vi "Graph_manipulations.vi"(0 "RF Slider in":cluster{i32, i32}, 1 "RF Slider 1":cluster{i32, i32}, 2 "Gaussian Noise SD":dbl, 5 "Array in":dbl[](array[numeric]), 7 "AFP Slider":cluster{i32, i32}, 9 "Zero ensemble in":dbl[](array[numeric]), 12 "rho+ in":dbl[](array[numeric]), 13 "rho0 in":dbl[](array[numeric]), 14 "rho- in":dbl[](array[numeric])) -> (4 "Q Graph":cluster{"Array":dbl[], "Array 2":dbl[]}, 6 "P Graph and Intensities and RF":cluster{"Array":dbl[], "Array":dbl[]}[](array[cluster]), 8 "Array out":cluster{dbl[], "Zero ensemble out":dbl[]}[](array[cluster]))   [LabVIEW 2018]
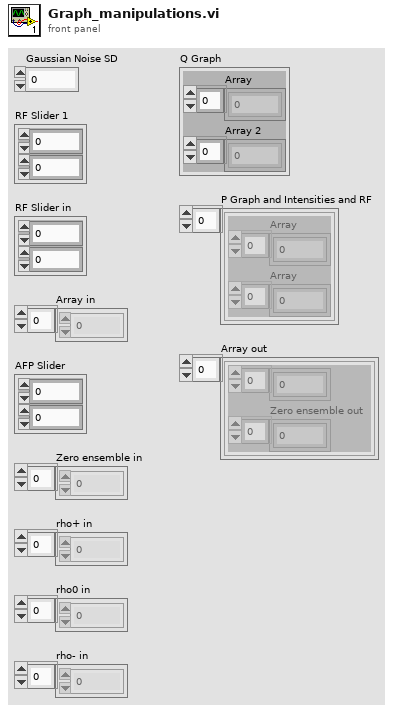
[diagram p1: front panel]
types:
  T1 = cluster{"Array in":dbl[], "Zero ensemble in":dbl[]}
  T2 = cluster{"Array in":dbl[], "Zero ensemble in":dbl[]}[]
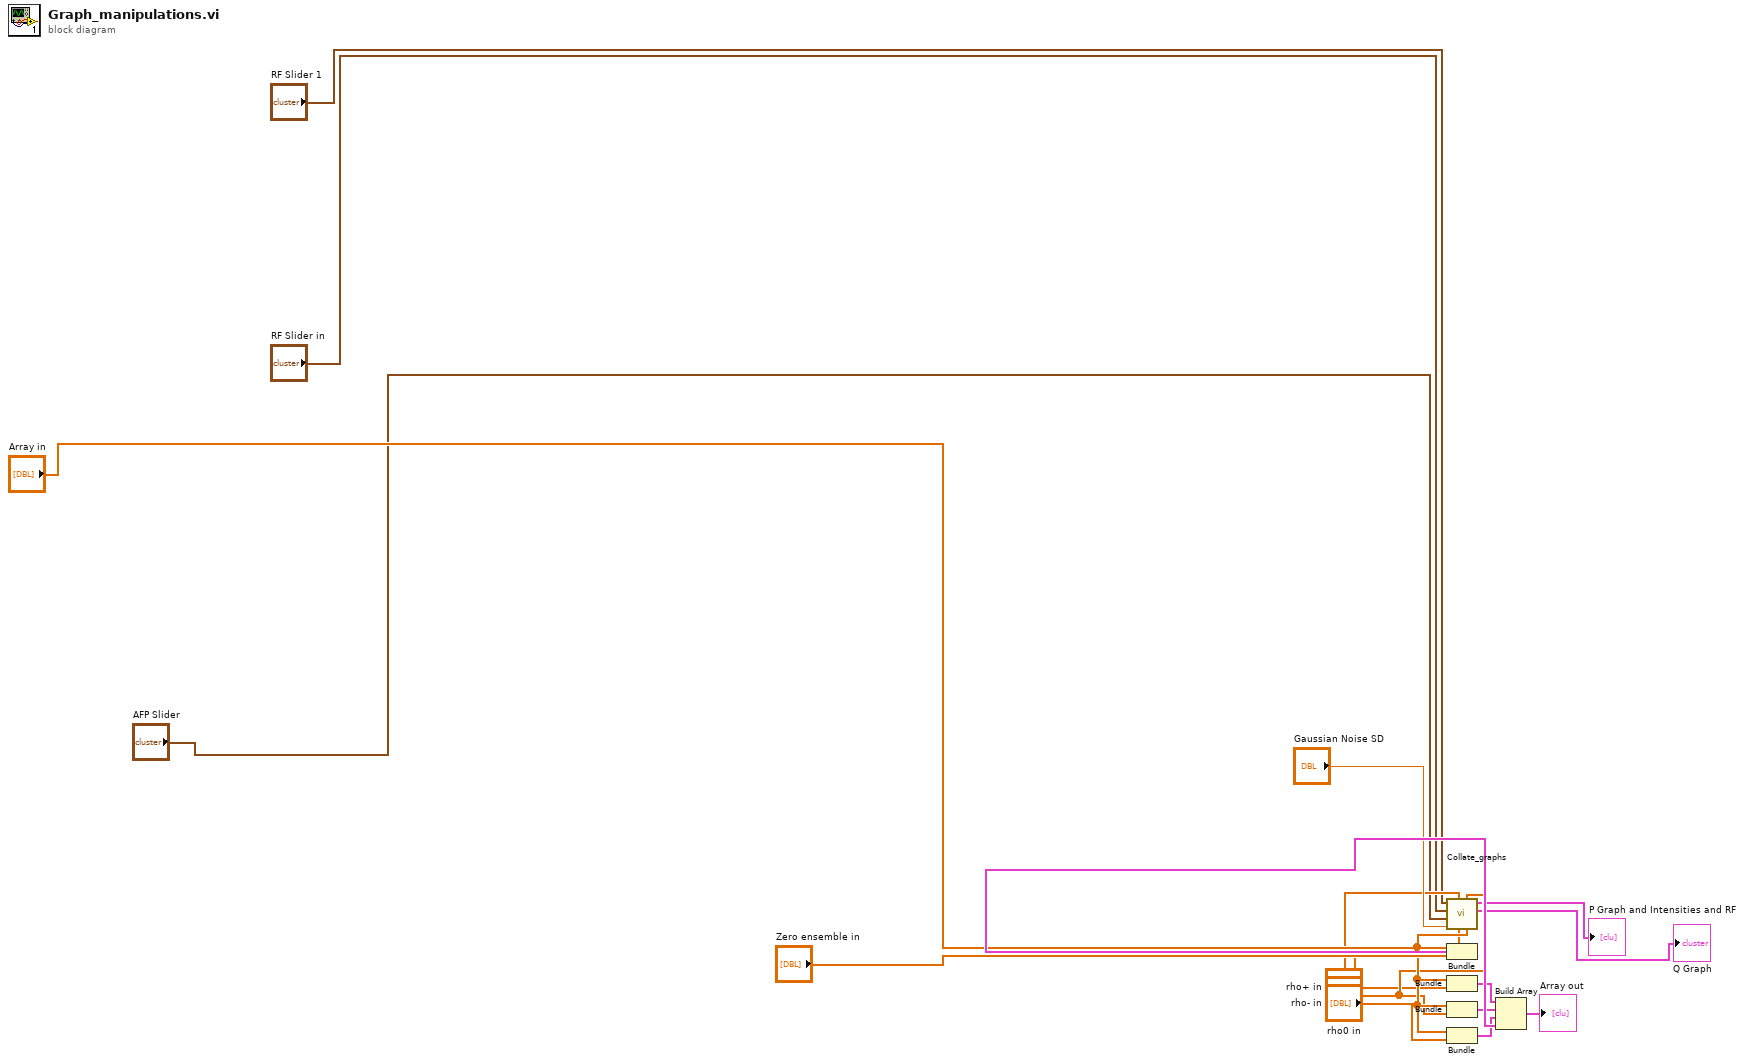
[diagram p0: block diagram]
diagram:
  n1 = call "Collate_graphs.vi"("R values"="Array in", "rho0"="rho0 in", "rho-"="rho- in", "rho+"="rho+ in", "Gaussian SD in"="Gaussian Noise SD", "AFP Range"="AFP Slider", "RF Range 2"="RF Slider in", "RF Range 1"="RF Slider 1") -> ("Q Graph"=→"Q Graph":cluster{"Array":dbl[], "Array 2":dbl[]}, "P Graph and Intensities and RF"=→"P Graph and Intensities and RF":cluster{"Array":dbl[], "Array":dbl[]}[])  [unwired: 2 in]
  n2 = Bundle("Array in"="Array in", "Zero ensemble in"="Zero ensemble in") -> (w15:T1)  [unwired: 1 in]
  n3 = Bundle("Array in"="Array in", "rho+ in"="rho+ in") -> (w7:cluster{"Array in":dbl[], "rho+ in":dbl[]})  [unwired: 1 in]
  n4 = Bundle("Array in"="Array in", "rho0 in"="rho0 in") -> (w6:cluster{"Array in":dbl[], "rho0 in":dbl[]})  [unwired: 1 in]
  n5 = Bundle("Array in"="Array in", "rho- in"="rho- in") -> (w8:cluster{"Array in":dbl[], "rho- in":dbl[]})  [unwired: 1 in]
  n6 = Build Array(w7, w6, w8, w15) -> (→"Array out":T2)
